vi "capt.vi"(6 "Graph in":cluster{dbl[], dbl[]}, 8 "error in":errorcluster, 9 "Length":i32=250, 11 "ON":bool) -> (0 "error out":errorcluster, 2 "Values":cluster{dbl[], dbl[]})   [LabVIEW 2013]
uses:
  GlobalVariables/CaptParameters.vi
  GlobalVariables/CommunicationActivity.vi
panel:
  in  "Address":u8=250
  in  "Channel":enum16{"CH0", "P1", "P2", "T", "TOB1", "TOB2"}(ring)=enum."P1"
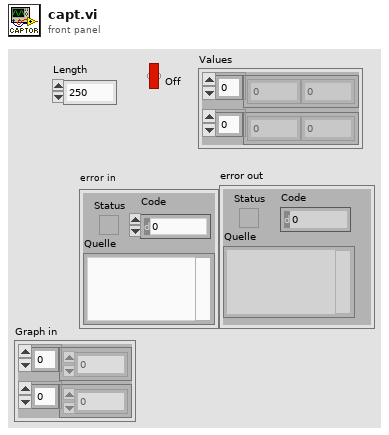
[diagram p1: front panel]
types:
  T1 = cluster{"SignalLoss":bool, "PumeActive":bool, "CaptorActive":bool}
  T2 = cluster{"SignalLoss":bool, "PumeActive":bool, bool}
  T3 = cluster{"baudrate":u32, "databits":u16, "paritybit":u16, "stopbits":u16, "flux control":u16, "Port":string, "Register Address":u16, "Serial Parameters":cluster{"Mode":enum16{"RTU", "ASCII"}, "Slave Address":u8}, "Timeout":u32}
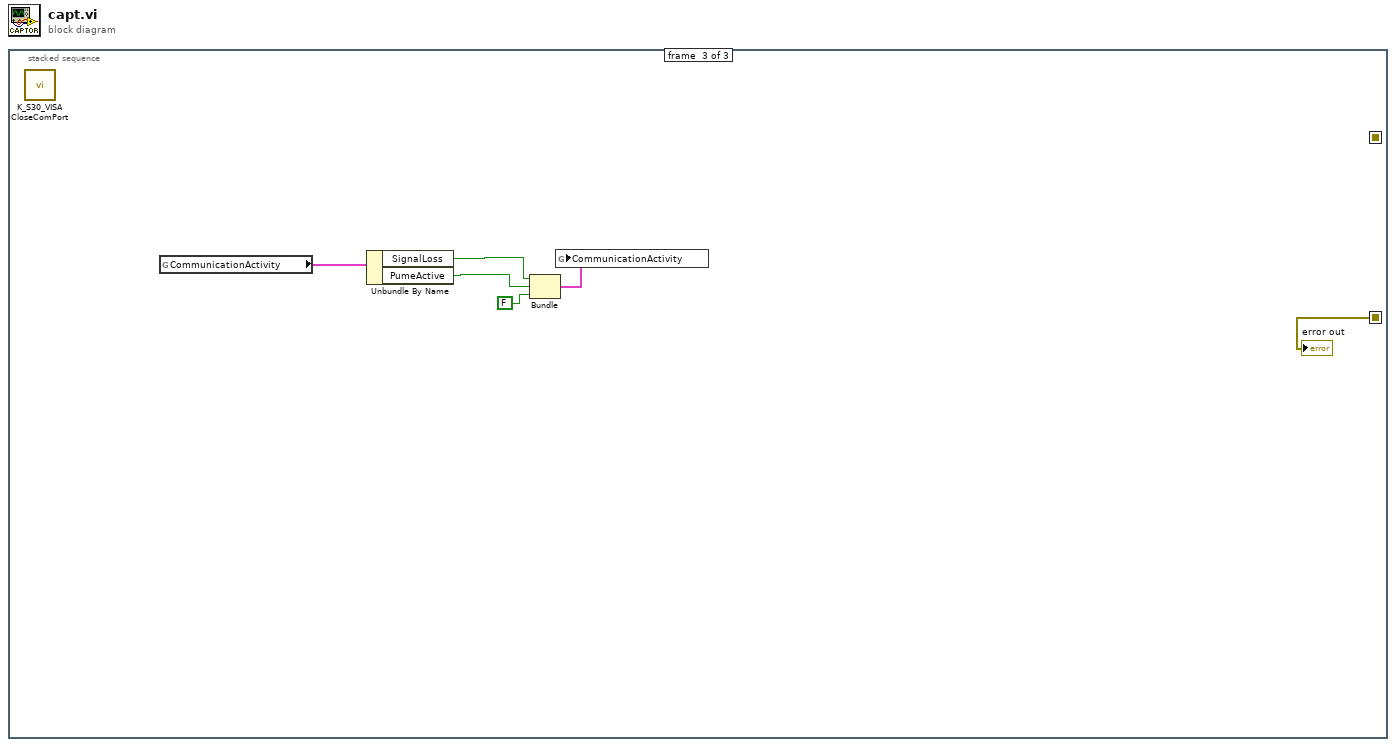
[diagram p0: block diagram]
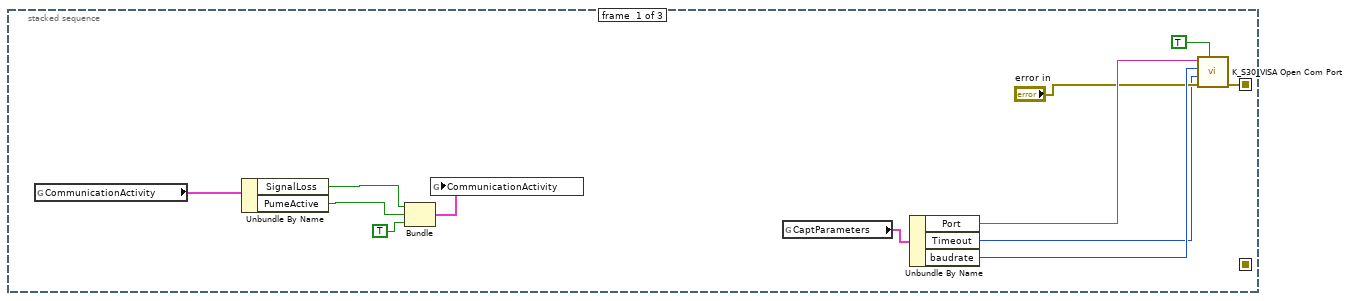
[diagram p2: hidden frame]
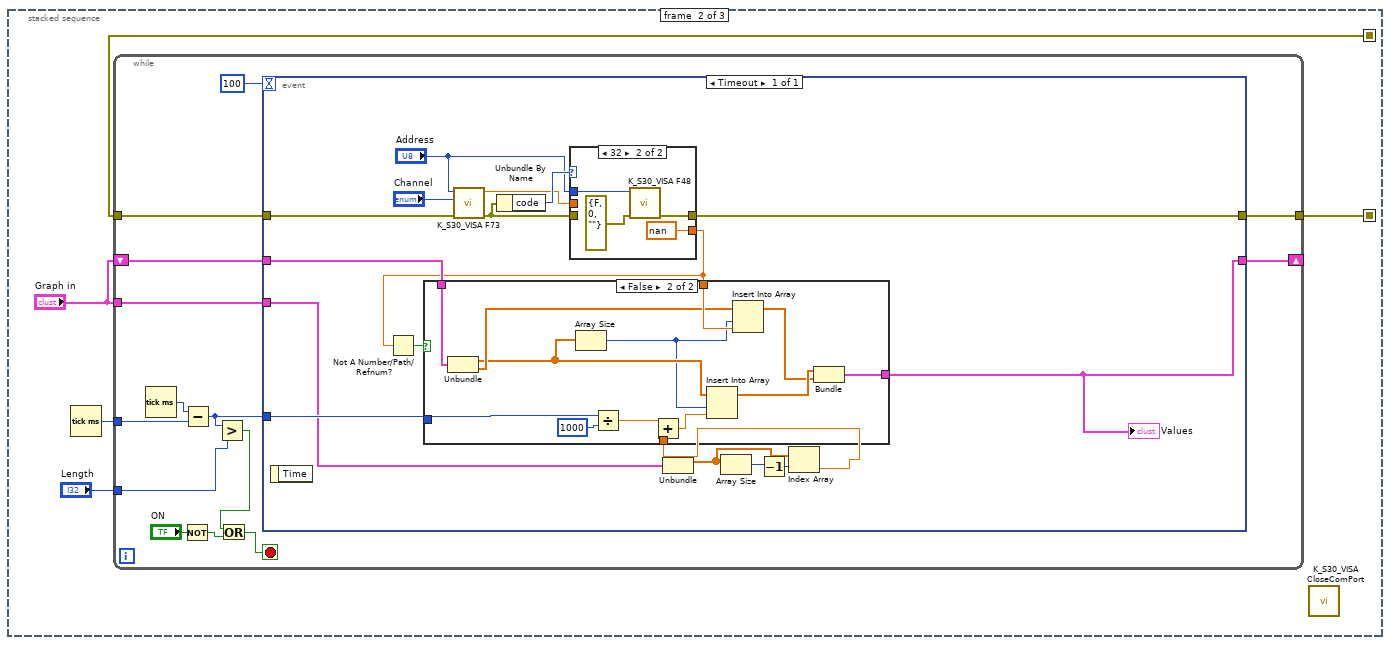
[diagram p3: hidden frame]
diagram:
  n1 = stacked-sequence {
    seq-local: [w11 _ _] -> [_ w15 _]
    seq-local: [_ w14 _] -> [_ _ w74]
    frame #0 {
      n2 = global read "CommunicationActivity.vi" "CommunicationActivity"() -> (w5:T1)
      n3 = Unbundle By Name(w5) -> ("SignalLoss"=w2:bool, "PumeActive"=w3:bool)
      n4 = Bundle("SignalLoss"=w2, "PumeActive"=w3, TRUE) -> (w4:T2)  [unwired: 1 in]
      n5 = global write "CommunicationActivity.vi" "CommunicationActivity"(w4) -> ()
      n6 = global read "CaptParameters.vi" "CaptParameters"() -> (w10:T3)
      n7 = Unbundle By Name(w10) -> ("Port"=w9:string, "Timeout"=w6:u32, "baudrate"=w8:u32)
      n8 = call "K_S30_VISA Open Com Port.vi"("RS-converter:\necho"=TRUE ("RS-converter: echo"), "error in (no error)"="error in", "timeout"=w6, "Baudrate"=w8, "VISA resource name"=w9) -> ("error out"=w11:errorcluster)  [unwired: 3 in, 1 out]
    }
    frame #1 {
      n9 = Tick Count (ms)() -> (millisecond timer value=w16:u32)
      n10 = while {
        tunnel: "Length" -> [w18]
        tunnel: w16 -> [w29]
        tunnel: w15 -> [w27]
        tunnel: [w26] -> w14
        shift-right: [w24] -> _
        shift-left: "Graph in" -> [w25]
        tunnel: "Graph in" -> [w19]
        stop <- w20 stop-if-true
        n11 = Tick Count (ms)() -> (millisecond timer value=w30:u32)
        n12 = Not(x="ON") -> (.not. x?=w22:bool)
        n13 = Subtract(x=w30, y=w29) -> (x-y=w28:u32)
        n14 = Greater?(x=w28, y=w18) -> (0:w21:bool)
        n15 = Or(x=w21, y=w22) -> (x .or. y?=w20:bool)
        n16 = event shown="[0] Timeout" {
          selector: _ -> [_]
          dyn-events: _ -> [_]
          timeout: 100 -> [_]
          tunnel: w28 -> [w48]
          tunnel: w27 -> [w47]
          tunnel: [w46] -> w26
          tunnel: w25 -> [w40]
          tunnel: [w39] -> w24
          tunnel: w19 -> [w38]
          event Timeout {
            n17 = event-data() -> ()  [unwired: 1 in, 1 out]
            n18 = call "K_S30_VISA F73.vi"("error in"=w47, "Channel"="Channel", "Address"="Address") -> ("error out"=w42:errorcluster, "Value"=w41:sgl)  [unwired: 2 in, 1 out]
            n19 = Unbundle By Name(w42) -> ("code"=w44:i32)
            n20 = case shown="32" w44 {
              tunnel: "Address" -> [_ w68]
              tunnel: w42 -> [w63 _]
              tunnel: w41 -> [w64 _]
              tunnel: [w64 sgl nan] -> w32
              tunnel: [w63 w66] -> w46
              frame 0, Default {
              }
              frame 32 {
                n21 = call "K_S30_VISA F48.vi"("error in"=errorcluster {"status"=FALSE, "code"=0, "source"=""}, "Address"=w68) -> ("error out"=w66:errorcluster)  [unwired: 3 in, 2 out]
              }
            }
            n22 = Not A Number/Path/Refnum?(number/path/refnum=w32) -> (NaN/Path/Refnum?=w33:bool)
            n23 = Unbundle(w38) -> (w35:dbl[])  [unwired: 1 out]
            n24 = Array Size(array=w35) -> (size(s)=w37:i32)
            n25 = Decrement(x=w37) -> (x-1=w36:i32)
            n26 = Index Array(array=w35, index=w36) -> (element=w34:dbl)
            n27 = case shown="False" w33 {
              tunnel: w48 -> [_ w62]
              tunnel: w32 -> [_ w60]
              tunnel: w40 -> [w49 w59]
              tunnel: [w49 w58] -> w39
              tunnel: w34 -> [_ w52]
              frame True {
              }
              frame False {
                n28 = Unbundle(w59) -> (w51:dbl[], w55:dbl[])
                n29 = Array Size(array=w51) -> (size(s)=w50:i32)
                n30 = Divide(x=w62, y=1000) -> (x/y=w54:dbl)
                n31 = Add(x=w54, y=w52) -> (x+y=w53:dbl)
                n32 = Insert Into Array(array=w51, index=w50, new element=w53) -> (w57:dbl[])
                n33 = Insert Into Array(array=w55, index=w50, new element=w60) -> (w56:dbl[])
                n34 = Bundle(w57, w56) -> (w58:cluster{dbl[], dbl[]})  [unwired: 1 in]
              }
            }
            "Values" <- w39
          }
        }
      }
      n35 = call "K_S30_VISA CloseComPort.vi"() -> ()  [unwired: 7 in, 1 out]
    }
    frame #2 {
      n36 = call "K_S30_VISA CloseComPort.vi"() -> ()  [unwired: 7 in, 1 out]
      n37 = global read "CommunicationActivity.vi" "CommunicationActivity"() -> (w73:T1)
      n38 = Unbundle By Name(w73) -> ("SignalLoss"=w70:bool, "PumeActive"=w71:bool)
      n39 = Bundle("SignalLoss"=w70, "PumeActive"=w71, FALSE) -> (w72:T2)  [unwired: 1 in]
      n40 = global write "CommunicationActivity.vi" "CommunicationActivity"(w72) -> ()
      "error out" <- w74
    }
  }
